vi "execute.vi"(8 "error in (no error)":errorcluster, 10 "SQL query":string, 11 "Database in":refnum<class "Database.lvclass">) -> (0 "error out":errorcluster, 3 "Database out":refnum<class "Database.lvclass">)   [LabVIEW 2018, in "Database.lvclass"]
uses:
  Database.lvclass
  Database.lvclass/Database.ctl
  <vilib>/addons/database/Connection.llb/Conn Execute.vi
  <vilib>/addons/database/Recordset.llb/Rec Destroy - Connection.vi
  <vilib>/addons/database/NI_Database_API.lvlib
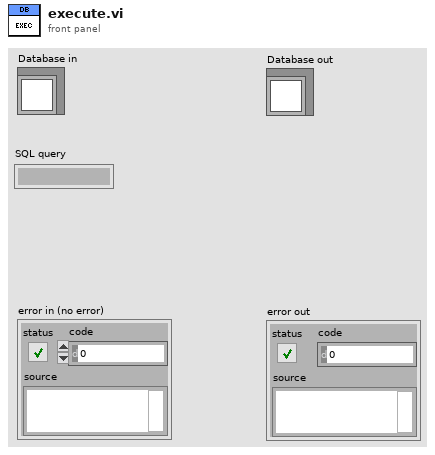
[diagram p1: front panel]
types:
  T1 = typedef "NI_Database_API.lvlib/Conn ObjectReference.ctl" = refnum<k1>
  T2 = typedef "NI_Database_API.lvlib/Rec ObjectReference.ctl" = refnum<k1>
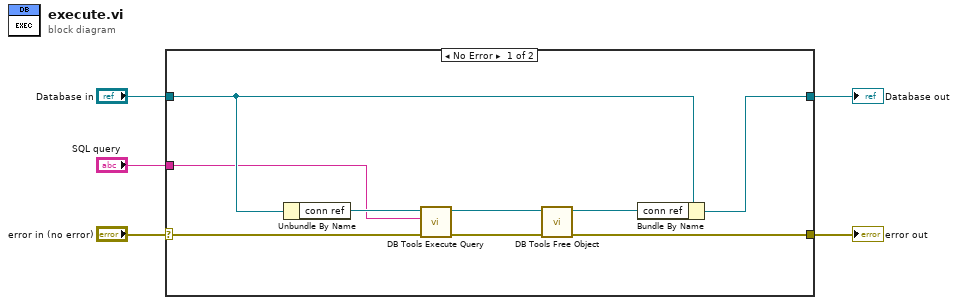
[diagram p0: block diagram]
diagram:
  n1 = case shown="No Error" "error in (no error)" {
    selector: "error in (no error)" -> [w9 w15]
    tunnel: [w14 w15] -> w5
    tunnel: [w13 w16] -> w4
    tunnel: "Database in" -> [w11 w16]
    tunnel: "SQL query" -> [w8 _]
    frame No Error {
      n2 = Unbundle By Name(w11) -> ("conn ref"=w10:T1)
      n3 = call-poly <vilib>:"DB Tools Execute Query.vi"("error in (no error)"=w9, "SQL query"=w8, "connection reference"=w10) -> ("error out"=w6:errorcluster, "recordset reference"=w7:T2)  [unwired: 2 in, 3 out]
      n4 = call-poly <vilib>:"DB Tools Free Object.vi"("error in (no error)"=w6, "recordset reference"=w7) -> ("error out"=w14:errorcluster, "connection reference"=w12:T1)  [unwired: 8 out]
      n5 = Bundle By Name(cluster=w11, "conn ref"=w12) -> (w13:refnum<class "Database.lvclass">)
    }
    frame Error {
    }
  }
  "error out" <- w5
  "Database out" <- w4
